vi "ge_EditBool.vi"(7 "ItemNames":string[][](array[string]), 8 "error in":errorcluster, 9 "Cell Val":string, 10 "Active Cell":T1, 11 "reference":refnum<vi>) -> (0 "error out":errorcluster, 1 "Discard?":bool)   [LabVIEW 2012]
uses:
  <vilib>/Utility/miscctls.llb/LVRowAndColumnTypeDef.ctl
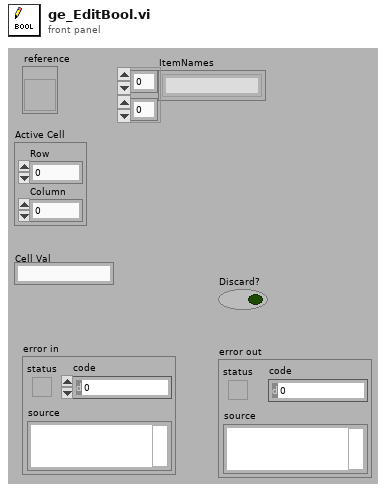
[diagram p1: front panel]
types:
  T1 = typedef "LVRowAndColumnTypeDef.ctl" = cluster{"Row":i32, "Column":i32}
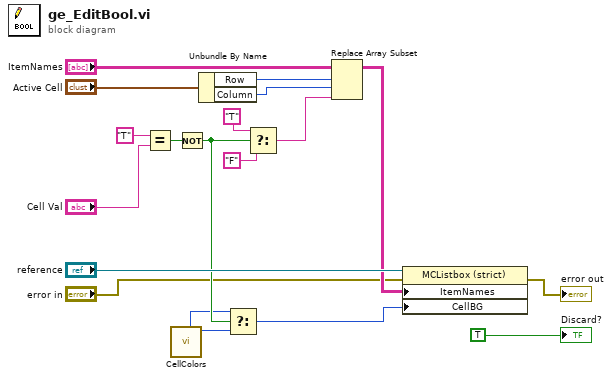
[diagram p0: block diagram]
diagram:
  n1 = Equal?(x="T" ("y"), y="Cell Val") -> (x = y?=w13:bool)
  n2 = call "CellColors.vi"() -> ("Normal"=w15:u32, "True"=w14:u32)  [unwired: 8 in, 2 out]
  n3 = Not(x=w13) -> (.not. x?=w17:bool)
  n4 = Unbundle By Name("Active Cell") -> ("Row"=w7:i32, "Column"=w8:i32)
  n5 = Select(t=w14, s=w17, f=w15) -> (s? t:f=w16:u32)
  n6 = Select(t="T" ("y"), s=w17, f="F" ("y")) -> (s? t:f=w9:string)
  n7 = Replace Array Subset(array="ItemNames", new element=w9, index (row)=w7, index (col)=w8) -> (w11:string[][])
  n8 = property class="MCListbox (strict)"(reference="reference", error in="error in", "ItemNames"=w11, "CellBG"=w16) -> (error out=→"error out":errorcluster)  [unwired: 1 out]
  "Discard?" <- TRUE ("Discard?")
